vi "5900PRSet_Obsolete.vi"(11 "ExitSendCmd":bool) -> (15 "no 5900?":bool)   [LabVIEW 2022 SP3]
doc: "This application VI allows the user to set the desired parameters in the \n5800 / 5900 P / R. just select thevalues that you want to set the instrument to from the 5800 / 5900 user interface and click on the send to 5800 button."
uses:
  ScanningControl/Motion Controllers/-MotionRoutines/MotionGlobals.vi
panel:
  out "ATTENUATORS(db)":dbl format="%.2f"
  in  "OUTPUT ATTENUATION":u16(ring) items=["00.0", "00.5", "01.0", "01.5", "02.0", "02.5", "03.0", "03.5", "04.0", "04.5", "05.0", "05.5", "06.0", "06.5", "07.0", "07.5", "08.0", "08.5", "09.0", "09.5", "10.0", "10.5", "11.0", "11.5", "12.0", "12.5", "13.0", "13.5", "14.0", "14.5", "15.0", "15.5"]
  in  "INPUT ATTENUATION":u16(ring) items=["00.0", "10.0", "20.0", "30.0", "40.0", "50.0"]
  in  "GAIN(db)":u16(ring) items=["26.0", "40.0", "54.0"]
  in  "PRF(KHz)":u16(ring)=1 items=["XREMT", "EXBNC", "0.200", "0.500", "1.000", "2.000", "5.000", "10.00", "20.00"]
  in  "MODE":u16(ring) items=["P/ E", "THRU", "RPP", "EXT_PLSR"]
  in  "LP FILT(IN MHz)":u16(ring) items=["20", "50", "100", "200"]
  in  "HP FILT(IN KHz)":u16(ring) items=["1", "1000", "3000", "10000"]
  in  "DAMPING (IN Ohm)":u16(ring) items=["7", "10", "16", "20", "26", "30", "40", "50"]
  in  "ENERGY(UJ)":u16(ring) items=["1", "2", "4", "8", "16", "32"]
  # "MODEL 5900"
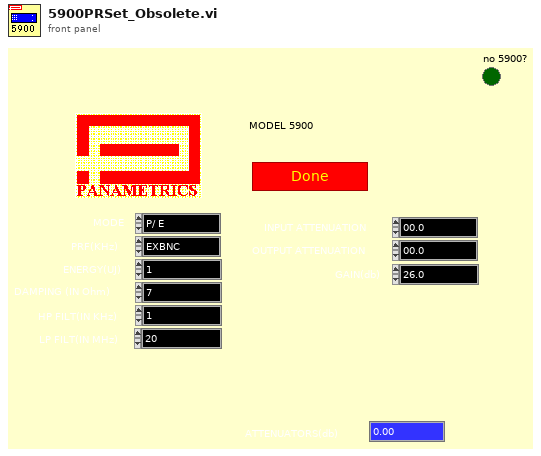
[diagram p1: front panel]
types:
  T1 = typedef "location.ctl" = enum16{"Automatic", "WCM Main", "Hawaii", "Columbia MM3000", "Columbia  NI System", "NYU", "RRI 2", "UHI Allen", "CUMC RT", "Chiba", "Stony Brook", "WCM Microscopy", "WCM Aeoretch", "WCM Optics Lab", "WCM Main 2Axis", "WCM Rotation", "WCM SAM SMAC", "SERI GP"}
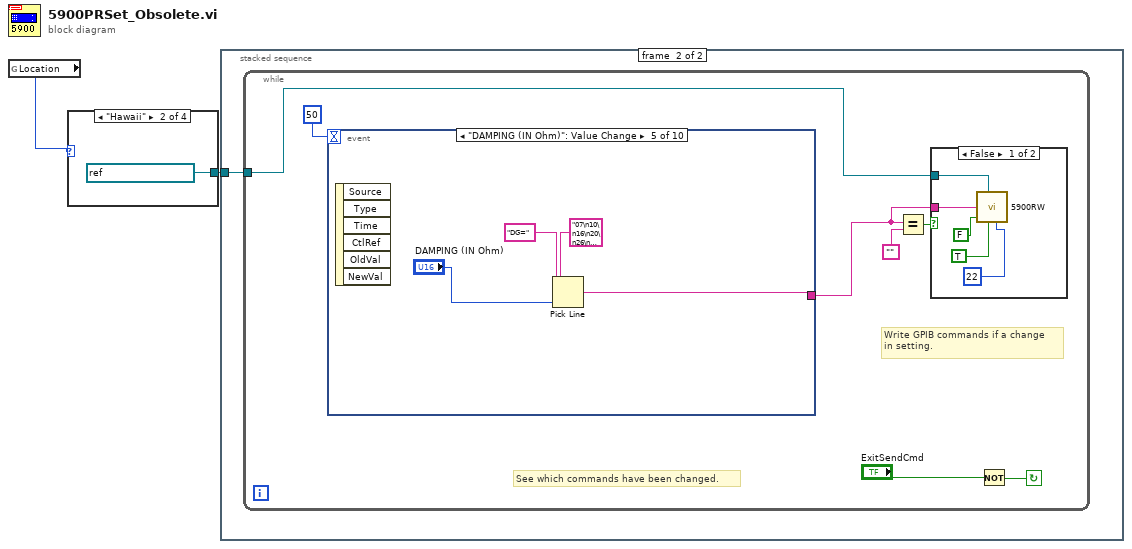
[diagram p0: block diagram]
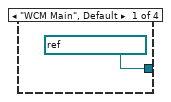
[diagram p2: hidden frame]
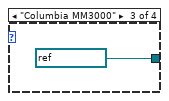
[diagram p3: hidden frame]
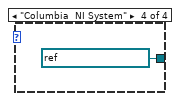
[diagram p4: hidden frame]
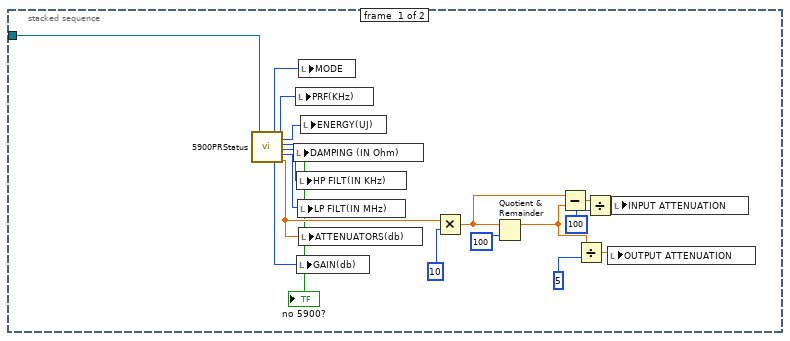
[diagram p5: hidden frame]
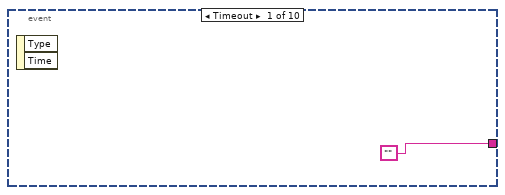
[diagram p7: hidden frame]
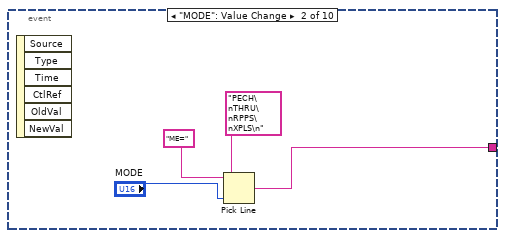
[diagram p8: hidden frame]
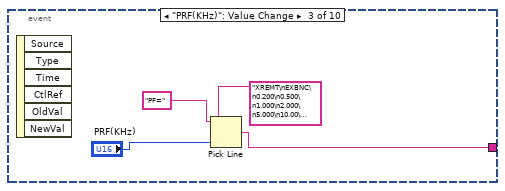
[diagram p9: hidden frame]
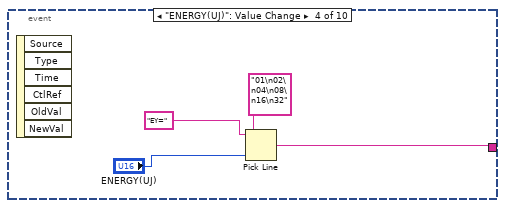
[diagram p10: hidden frame]
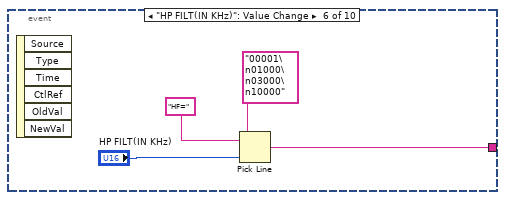
[diagram p11: hidden frame]
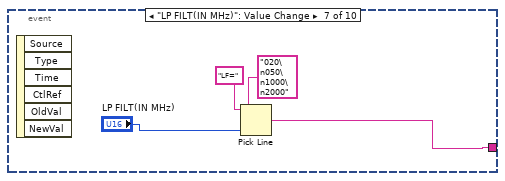
[diagram p12: hidden frame]
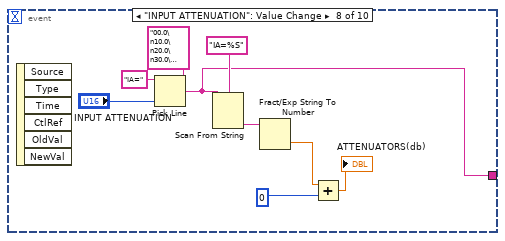
[diagram p13: hidden frame]
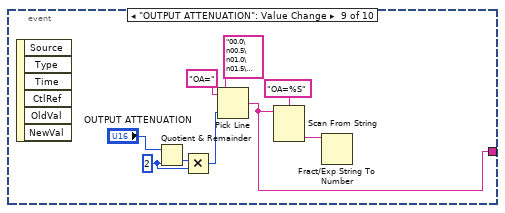
[diagram p14: hidden frame]
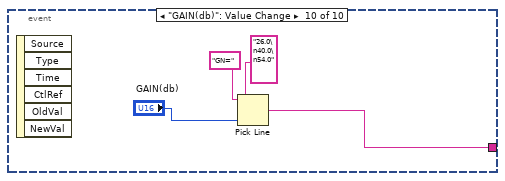
[diagram p15: hidden frame]
diagram:
  n1 = global read "MotionGlobals.vi" "Location"() -> (w1:T1)
  n2 = case shown="\"Hawaii\"" w1 {
    tunnel: [refnum<visa-resource-name> "GPIB::1::INSTR" ("VISA resource name") refnum<visa-resource-name> "GPIB1::1::INSTR" ("VISA resource name") refnum<visa-resource-name> "GPIB0::9" ("VISA resource name") refnum<visa-resource-name> "GPIB0::9::INSTR" ("VISA resource name")] -> w2
    frame "WCM Main", Default {
    }
    frame "Hawaii" {
    }
    frame "Columbia MM3000" {
    }
    frame "Columbia  NI System" {
    }
  }
  n3 = stacked-sequence {
    tunnel: w2 -> [w9 w26]
    frame #0 {
      n4 = call "5900PRStatus.vi"("VISA resource name"=w9) -> ("no 5900?"=→"no 5900?":bool, "MODE"=w25:u8, "GAIN(db)"=w19:u8, "PRF(KHz)"=w24:i8, "ENERGY(UJ)"=w23:u8, "DAMPING (IN Ohm)"=w22:u8, "HP FILT(IN KHz)"=w21:u8, "LP FILT(IN MHz)"=w20:u8, "ATTENUATORS(db)"=w8:dbl)  [unwired: 10 out]
      n5 = local write "DAMPING (IN Ohm)"(w22) -> ()
      n6 = local write "PRF(KHz)"(w24) -> ()
      n7 = local write "HP FILT(IN KHz)"(w21) -> ()
      n8 = local write "GAIN(db)"(w19) -> ()
      n9 = local write "LP FILT(IN MHz)"(w20) -> ()
      n10 = local write "MODE"(w25) -> ()
      n11 = local write "ATTENUATORS(db)"(w8) -> ()
      n12 = local write "ENERGY(UJ)"(w23) -> ()
      n13 = Multiply(x=w8, y=10) -> (x*y=w17:dbl)
      n14 = Quotient & Remainder(x=w17, y=100) -> (x-y*floor(x/y)=w13:dbl)  [unwired: 1 out]
      n15 = Subtract(x=w17, y=w13) -> (x-y=w16:dbl)
      n16 = Divide(x=w13, y=5) -> (x/y=w15:dbl)
      n17 = Divide(x=w16, y=100) -> (x/y=w14:dbl)
      n18 = local write "OUTPUT ATTENUATION"(w15) -> ()
      n19 = local write "INPUT ATTENUATION"(w14) -> ()
    }
    frame #1 {
      n20 = while {
        tunnel: w26 -> [w31]
        stop <- w33 continue-if-true
        # "Write GPIB commands if a change\nin setting."
        # "See which commands have been changed."
        n21 = event shown="[4] \"DAMPING (IN Ohm)\": Value Change" {
          selector: _ -> [_ _ _ _ _ _ _ _ _ _]
          dyn-events: _ -> [_ _ _ _ _ _ _ _ _ _]
          timeout: 50 -> [_ _ _ _ _ _ _ _ _ _]
          tunnel: ["" w40 w44 w48 w52 w56 w60 w65 w74 w82] -> w29
          event Timeout {
            n22 = event-data() -> ()  [unwired: 3 out]
          }
          event "MODE": Value Change {
            n23 = event-data() -> ()  [unwired: 7 out]
            n24 = Pick Line(string ("")="ME=", multi-line string="PECH\nTHRU\nRPPS\nXPLS\n", line index="MODE") -> (output string=w40:string)
          }
          event "PRF(KHz)": Value Change {
            n25 = event-data() -> ()  [unwired: 7 out]
            n26 = Pick Line(string ("")="PF=", multi-line string="XREMT\nEXBNC\n0.200\n0.500\n1.000\n2.000\n5.000\n10.00\n20.00\n", line index="PRF(KHz)") -> (output string=w44:string)
          }
          event "ENERGY(UJ)": Value Change {
            n27 = event-data() -> ()  [unwired: 7 out]
            n28 = Pick Line(string ("")="EY=", multi-line string="01\n02\n04\n08\n16\n32", line index="ENERGY(UJ)") -> (output string=w48:string)
          }
          event "DAMPING (IN Ohm)": Value Change {
            n29 = event-data() -> ()  [unwired: 7 out]
            n30 = Pick Line(string ("")="DG=", multi-line string="07\n10\n16\n20\n26\n30\n40\n50\n", line index="DAMPING (IN Ohm)") -> (output string=w52:string)
          }
          event "HP FILT(IN KHz)": Value Change {
            n31 = event-data() -> ()  [unwired: 7 out]
            n32 = Pick Line(string ("")="HF=", multi-line string="00001\n01000\n03000\n10000", line index="HP FILT(IN KHz)") -> (output string=w56:string)
          }
          event "LP FILT(IN MHz)": Value Change {
            n33 = event-data() -> ()  [unwired: 7 out]
            n34 = Pick Line(string ("")="LF=", multi-line string="020\n050\n1000\n2000", line index="LP FILT(IN MHz)") -> (output string=w60:string)
          }
          event "INPUT ATTENUATION": Value Change {
            n35 = event-data() -> ()  [unwired: 7 out]
            n36 = Pick Line(string ("")="IA=", multi-line string="00.0\n10.0\n20.0\n30.0\n40.0\n50.0\n60.0", line index="INPUT ATTENUATION") -> (output string=w65:string)
            n37 = Scan From String(format string="IA=%S", input string=w65) -> (output 1=w67:string)  [unwired: 2 in, 4 out]
            n38 = Fract/Exp String To Number(string=w67) -> (number=w71:dbl)  [unwired: 4 out]
            n39 = Add(x=w71, y=0) -> (x+y=→"ATTENUATORS(db)":dbl)
          }
          event "OUTPUT ATTENUATION": Value Change {
            w76 = 2
            n40 = event-data() -> ()  [unwired: 7 out]
            n41 = Quotient & Remainder(x="OUTPUT ATTENUATION", y=w76) -> (floor(x/y)=w77:i32)  [unwired: 1 out]
            n42 = Multiply(x=w77, y=w76) -> (x*y=w78:i32)
            n43 = Pick Line(string ("")="OA=", multi-line string="00.0\n00.5\n01.0\n01.5\n02.0\n02.5\n03.0\n03.5\n04.0\n04.5\n05.0\n05.5\n06.0\n06.5\n07.0\n07.5\n08.0\n08.5\n09.0\n09.5\n10.0\n10.5\n11.0\n11.5\n12.0\n12.5\n13.0\n13.5\n14.0\n14.5\n15.0\n15.5", line index=w78) -> (output string=w74:string)
            n44 = Scan From String(format string="OA=%S", input string=w74) -> (output 1=w75:string)  [unwired: 2 in, 4 out]
            n45 = Fract/Exp String To Number(string=w75) -> ()  [unwired: 5 out]
          }
          event "GAIN(db)": Value Change {
            n46 = event-data() -> ()  [unwired: 7 out]
            n47 = Pick Line(string ("")="GN=", multi-line string="26.0\n40.0\n54.0", line index="GAIN(db)") -> (output string=w82:string)
          }
        }
        n48 = Equal?(x=w29, y="") -> (x = y?=w28:bool)
        n49 = case shown="False" w28 {
          tunnel: w29 -> [w38 _]
          tunnel: w31 -> [w35 _]
          frame False {
            n50 = call "5900RW.vi"("VISA resource name"=w35, "ENTER STRING"=w38, "Read ?"=FALSE, "Write ?"=TRUE, "# bytes\nto read"=22) -> ()  [unwired: 5 out]
          }
          frame True {
          }
        }
        n51 = Not(x="ExitSendCmd") -> (.not. x?=w33:bool)
      }
    }
  }
